vi "show_mouse_position.vi"() -> ()   [LabVIEW 2018]
uses:
  User32.dll
panel:
  in  "stop":bool
  out "position":cluster{i32, i32}
  out "error out 2":errorcluster
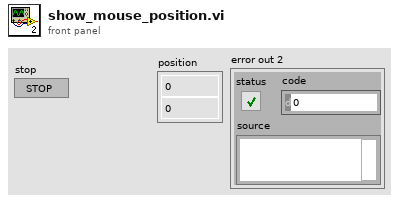
[diagram p1: front panel]
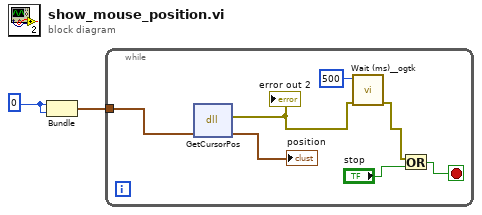
[diagram p0: block diagram]
diagram:
  w2 = 0
  n1 = Bundle(w2, w2) -> (w1:cluster{i32, i32})  [unwired: 1 in]
  n2 = while {
    tunnel: w1 -> [w8]
    stop <- w7 stop-if-true
    n3 = dll-call lib="User32.dll" fn="GetCursorPos"("position"=w8) -> (error out=w4:errorcluster, "position"=→"position":cluster{i32, i32})  [unwired: 4 in, 1 out]
    "error out 2" <- w4
    n4 = call <userlib>:"Wait (ms)__ogtk.vi"("error in (no error)"=w4, "milliseconds to wait"=u32 500) -> ("error out"=w3:errorcluster)  [unwired: 8 in, 1 out]
    n5 = Or(x=w3, y="stop") -> (x .or. y?=w7:bool)
  }
